vi "close.vi"(8 "error in":errorcluster, 11 "J1939 runtime in":refnum<class "J1939 runtime.lvclass">) -> (0 "error out":errorcluster)   [LabVIEW 2013, in "J1939 runtime.lvclass"]
doc: "Provides an interface for terminating a module instance. While this interface performs no operations, a child should close and deallocate any open references or memory."
uses:
  J1939 runtime.lvclass
  J1939 runtime.lvclass/J1939 runtime.ctl
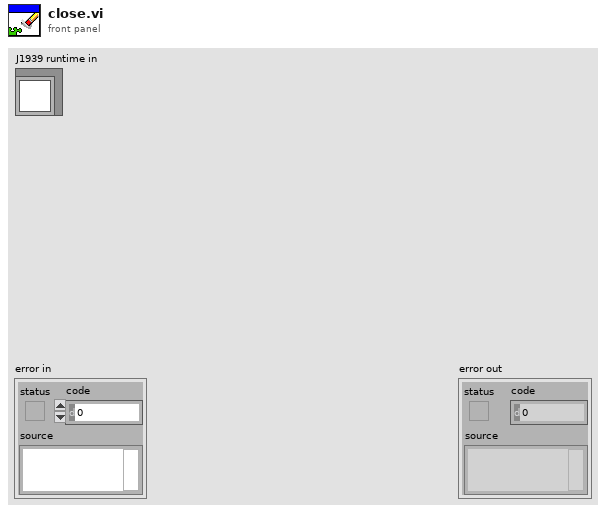
[diagram p1: front panel]
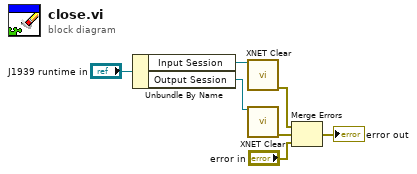
[diagram p0: block diagram]
diagram:
  n1 = Unbundle By Name("J1939 runtime in") -> ("Input Session"=w6:refnum<k21>, "Output Session"=w5:refnum<k21>)
  n2 = call <vilib>:"XNET Clear.vi"("session in"=w6) -> ("error out"=w2:errorcluster)  [unwired: 14 in]
  n3 = call <vilib>:"XNET Clear.vi"("session in"=w5) -> ("error out"=w1:errorcluster)  [unwired: 14 in]
  n4 = Merge Errors(w2, w1, "error in") -> (→"error out":errorcluster)
